vi "add_int16_roslv.vi"   [LabVIEW 2014]
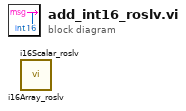
[diagram p0: block diagram]
diagram:
  n1 = call "i16Array_roslv.vi"() -> ()  [unwired: 5 in, 1 out]
  n2 = call "i16Scalar_roslv.vi"() -> ()  [unwired: 5 in, 1 out]
